vi "_PC_Pub_Sort2DArray.vi"(1 "Sort By":i32=1, 2 "Array":dbl[][](array[numeric])) -> (0 "transposed array":dbl[][](array[numeric]))   [LabVIEW 2018]
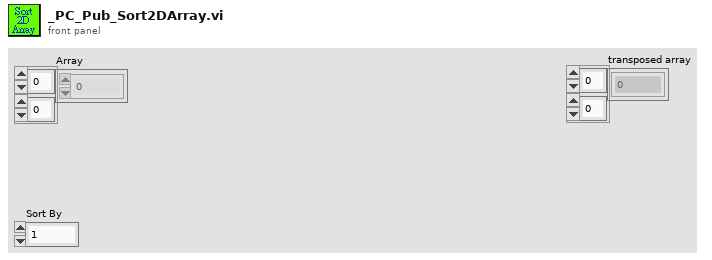
[diagram p1: front panel]
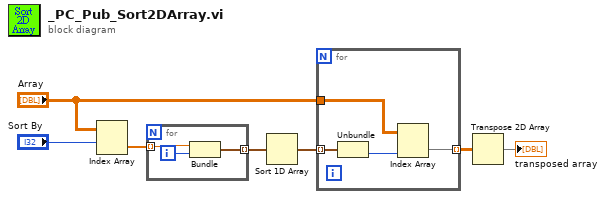
[diagram p0: block diagram]
diagram:
  n1 = Index Array(array="Array", index (row)="Sort By") -> (element=w6:dbl[])  [unwired: 1 in]
  n2 = for {
    tunnel: w6 -> [w10] mode=indexing
    tunnel: [w8] -> w5 mode=indexing
    i -> [w9]
    n3 = Bundle("number: 0 to 1"=w10, w9) -> (w8:cluster{"number: 0 to 1":dbl, i32})  [unwired: 1 in]
  }
  n4 = Sort 1D Array(array=w5) -> (sorted array=w4:cluster{"number: 0 to 1":dbl, i32}[])
  n5 = for {
    tunnel: "Array" -> [w14]
    tunnel: w4 -> [w13] mode=indexing
    tunnel: [w11] -> w3 mode=indexing
    n6 = Unbundle(w13) -> (w12:i32)  [unwired: 1 out]
    n7 = Index Array(array=w14, index (col)=w12) -> (element=w11:dbl[])  [unwired: 1 in]
  }
  n8 = Transpose 2D Array(2D array=w3) -> (transposed array=→"transposed array":dbl[][])
